vi "Acquisition Timer.vi"(10 "Minimum Loop Rate (Ticks)":u8=10, 11 "Loop Time (Ticks)":u32) -> (3 "Actual Time (Ticks)":u32)   [LabVIEW 2014]
doc: "This VI controls the timing for the FPGA write loop. The two inputs allow you to set a minimum rate, and then allow the user to decimate that rate slower should they desire. Use the Minimum Rate (Ticks) input to control the minimum loop rate. Use the Additional Time input to add in additional time between subsequent loop iterations."
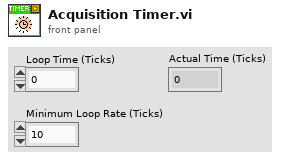
[diagram p1: front panel]
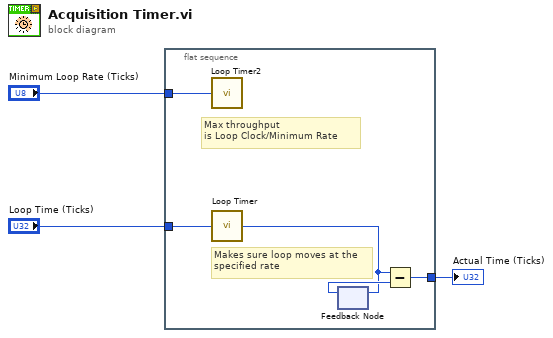
[diagram p0: block diagram]
diagram:
  n1 = flat-sequence {
    tunnel: "Loop Time (Ticks)" -> [w8]
    tunnel: [w5] -> w3
    tunnel: "Minimum Loop Rate (Ticks)" -> [w4]
    frame #0 {
      # "Max throughput\nis Loop Clock/Minimum Rate"
      # "Makes sure loop moves at the\nspecified rate"
      n2 = call "Loop Timer2"("Count(uSec)"=w4) -> ()  [unwired: 1 out]
      n3 = call "Loop Timer"("Count(Ticks)"=w8) -> ("Tick Count(Ticks)"=w6:u32)
      n4 = feedback-in #1(w6) -> ()
      n5 = feedback #1() -> (w7:u32)  [unwired: 1 out]
      n6 = Subtract(x=w6, y=w7) -> (x-y=w5:u32)
    }
  }
  "Actual Time (Ticks)" <- w3
